vi "Keithley 2450 Digitized Sweep.vi"() -> ()   [LabVIEW 2023]
doc: "Configure the sweep with the amplitude, source settings and takes current and voltage reading.\n\nNote:\nThis VI is applicable only to 2461 model."
uses:
  Keithley 2450.lvlib
  Public/Data/Read (Multiple Points).vi
panel:
  in  "Limit Level (0.1)":dbl=0.1
  in  "Delay (0) in Sec":dbl
  in  "Sample Rate (1000Hz)":u32=2500
  in  "Sweep Points":T1={"Start "=0.0, "Stop "=5.0, "Number of Points (5)"=100}
  in  "Source Mode  (0: Voltage)":u16(ring) items=["Voltage", "Current"]
  in  "VISA resource name":refnum<visa-resource-name>
  out "Waveform Graph":dbl[][](graph)=[[-0.0001858189, 0.007417283, 0.03360542, 0.04403445, 0.04793108, 0.04931186, 0.04991157, 0.05009001, 0.050169, 0.05021289, 0.05022166, 0.0502948, 0.05017778, 0.0501924, 0.05012805, 0.05020703, 0.05027724, 0.05013097, 0.05005784, 0.05013682, 0.05028309, 0.05022166, 0.05016023, 0.05013682, 0.05026846, 0.05003736, 0.05026846, 0.05008124, 0.04967754, 0.06964044, 0.08971742, 0.09662428, 0.09915767, 0.1002605, 0.1006028, 0.1006964, 0.1009071, 0.1008047, 0.1007023, 0.1006935, 0.10079, 0.1007959, 0.1007725, 0.1007988, 0.100673, 0.1007198, 0.1008105, 0.1007052, 0.1007257, 0.1006584, 0.1006935, 0.1007754, 0.1007754, 0.1007637, 0.1007052, 0.1005882, 0.1131528, 0.1376734, 0.146435, 0.1495388, 0.1505656, 0.1511127, 0.1512063, 0.1512092, 0.1511624, 0.151139, 0.1511624, 0.1513233, 0.1511917, 0.1512999, 0.1512005, 0.151256, 0.1513321, 0.1512209, 0.1512239, 0.1510981, 0.1511624, 0.1513233, 0.1512472, 0.1512999, 0.1512999, 0.1513496, 0.151256, 0.1512999, 0.1734568, 0.1922818, 0.1985187, 0.2007771, 0.2015465, 0.2017893, 0.2019765, 0.2018595, 0.201842, 0.2017601, 0.2017893, 0.2019063, 0.2018215, 0.2016898, 0.2017103, 0.2018069], [-0.0001858189, 0.007417283, 0.03360542, 0.04403445, 0.04793108, 0.04931186, 0.04991157, 0.05009001, 0.050169, 0.05021289, 0.05022166, 0.0502948, 0.05017778, 0.0501924, 0.05012805, 0.05020703, 0.05027724, 0.05013097, 0.05005784, 0.05013682, 0.05028309, 0.05022166, 0.05016023, 0.05013682, 0.05026846, 0.05003736, 0.05026846, 0.05008124, 0.04967754, 0.06964044, 0.08971742, 0.09662428, 0.09915767, 0.1002605, 0.1006028, 0.1006964, 0.1009071, 0.1008047, 0.1007023, 0.1006935, 0.10079, 0.1007959, 0.1007725, 0.1007988, 0.100673, 0.1007198, 0.1008105, 0.1007052, 0.1007257, 0.1006584, 0.1006935, 0.1007754, 0.1007754, 0.1007637, 0.1007052, 0.1005882, 0.1131528, 0.1376734, 0.146435, 0.1495388, 0.1505656, 0.1511127, 0.1512063, 0.1512092, 0.1511624, 0.151139, 0.1511624, 0.1513233, 0.1511917, 0.1512999, 0.1512005, 0.151256, 0.1513321, 0.1512209, 0.1512239, 0.1510981, 0.1511624, 0.1513233, 0.1512472, 0.1512999, 0.1512999, 0.1513496, 0.151256, 0.1512999, 0.1734568, 0.1922818, 0.1985187, 0.2007771, 0.2015465, 0.2017893, 0.2019765, 0.2018595, 0.201842, 0.2017601, 0.2017893, 0.2019063, 0.2018215, 0.2016898, 0.2017103, 0.2018069]]
  # "(c) 2021 National Instruments.  ALL RIGHTS RESERVED."
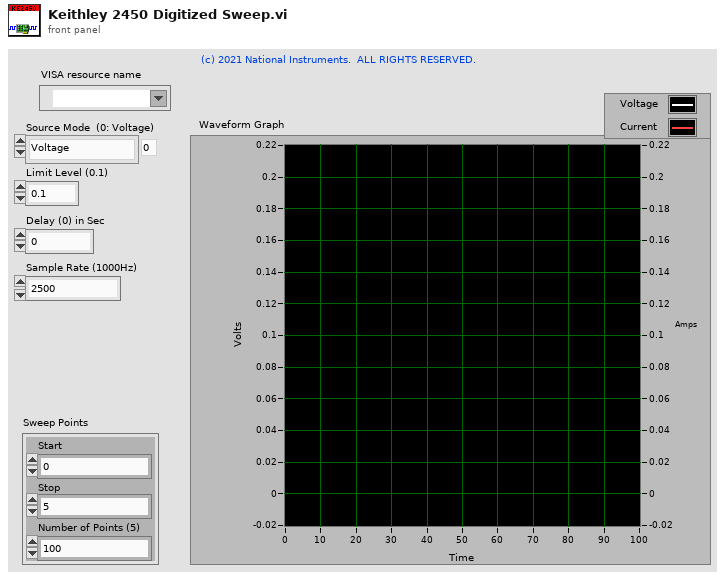
[diagram p1: front panel]
types:
  T1 = cluster{"Start ":dbl, "Stop ":dbl, "Number of Points (5)":u32}
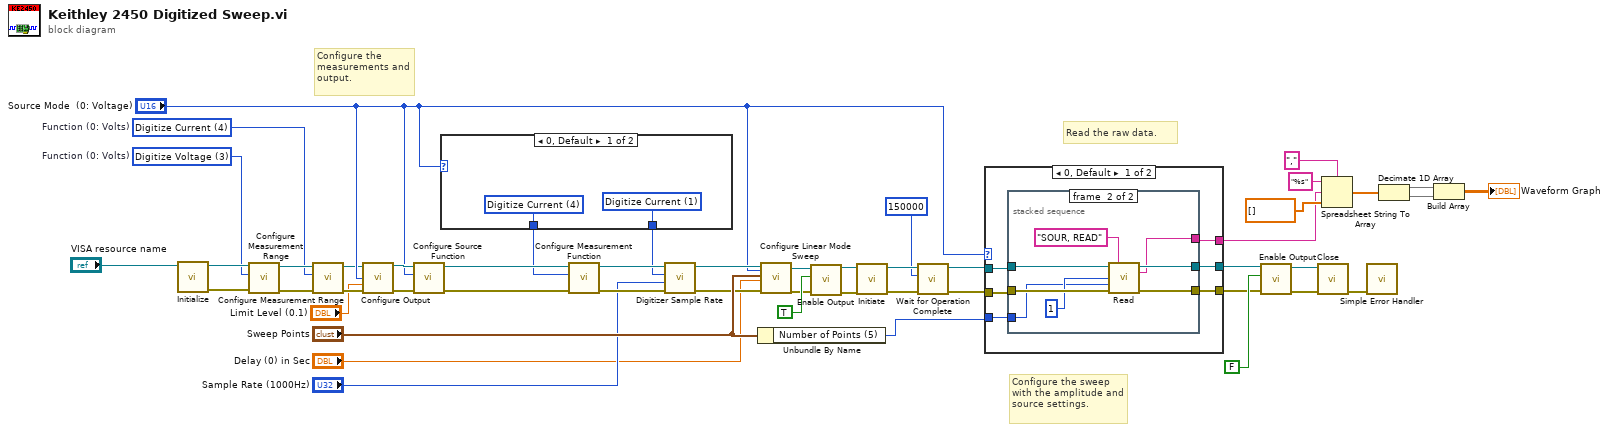
[diagram p0: block diagram]
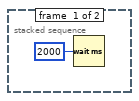
[diagram p2: hidden frame]
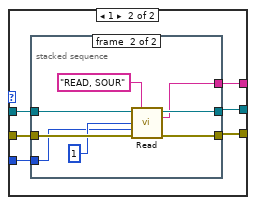
[diagram p3: hidden frame]
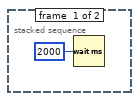
[diagram p4: hidden frame]
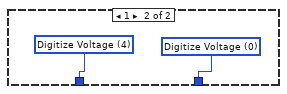
[diagram p5: hidden frame]
diagram:
  w6 = u16 4 items=["Volts", "Current", "Resistance", "Digitize Voltage", "Digitize Current"]  # Function (0: Volts)
  w7 = u16 3 items=["Volts", "Current", "Resistance", "Digitize Voltage", "Digitize Current"]  # Function (0: Volts)
  # "Read the raw data."
  # "Configure the sweep with the amplitude and source settings."
  # "Configure the measurements and output."
  n1 = call "Initialize.vi"("VISA resource name"="VISA resource name") -> ("error out"=w12:errorcluster, "VISA resource name out"=w13:refnum<visa-resource-name>)  [unwired: 9 in]
  n2 = call "Configure Measurement Range.vi"("error in (no error)"=w12, "Function (0: Volts)"=w7, "VISA resource name"=w13) -> ("error out"=w10:errorcluster, "VISA resource name out"=w11:refnum<visa-resource-name>)  [unwired: 7 in]
  n3 = call "Configure Measurement Range.vi"("error in (no error)"=w10, "Function (0: Volts)"=w6, "VISA resource name"=w11) -> ("error out"=w8:errorcluster, "VISA resource name out"=w9:refnum<visa-resource-name>)  [unwired: 7 in]
  n4 = call "Configure Output.vi"("VISA resource name"=w9, "Source Mode  (0: Voltage)"="Source Mode  (0: Voltage)", "Source Limit Level (0.1)"="Limit Level (0.1)", "error in (no error)"=w8) -> ("VISA resource name out"=w42:refnum<visa-resource-name>, "error out"=w43:errorcluster)  [unwired: 10 in]
  n5 = call "Configure Source Function.vi"("error in (no error)"=w43, "Function (0: Volts)"="Source Mode  (0: Voltage)", "VISA resource name"=w42) -> ("error out"=w25:errorcluster, "VISA resource name out"=w26:refnum<visa-resource-name>)  [unwired: 7 in]
  n6 = case shown="0, Default" "Source Mode  (0: Voltage)" {
    tunnel: [w51 w53] -> w5
    tunnel: [w50 w52] -> w4
    frame 0, Default {
      w50 = u16 1 items=["Digitize Voltage", "Digitize Current"] ("Function (0: Volts)")
      w51 = u16 4 items=["Voltage", "Current", "Resistance", "Digitize Voltage", "Digitize Current"] ("Function (0: Volts)")
    }
    frame 1 {
      w52 = u16 0 items=["Digitize Voltage", "Digitize Current"] ("Function (0: Volts)")
      w53 = u16 4 items=["Voltage", "Current", "Auto Resistance", "Manual Resistance", "Digitize Voltage", "Digitize Current"] ("Function (0: Volts)")
    }
  }
  n7 = call "Configure Measurement Function.vi"("error in (no error)"=w25, "Function (0: Volts)"=w5, "VISA resource name"=w26) -> ("error out"=w17:errorcluster, "VISA resource name out"=w18:refnum<visa-resource-name>)  [unwired: 7 in]
  n8 = call "Digitizer Sample Rate.vi"("error in (no error)"=w17, "Sample Rate (100000)"="Sample Rate (1000Hz)", "Digitize Function (Voltage)"=w4, "VISA resource name"=w18) -> ("error out"=w15:errorcluster, "VISA resource name out"=w16:refnum<visa-resource-name>)  [unwired: 6 in]
  n9 = Unbundle By Name("Sweep Points") -> ("Number of Points (5)"=w20:u32)
  n10 = call "Configure Linear Mode Sweep.vi"("VISA resource name"=w16, "Source Mode  (0: Voltage)"="Source Mode  (0: Voltage)", "Sweep Points"="Sweep Points", "Delay (0)"="Delay (0) in Sec", "error in (no error)"=w15) -> ("VISA resource name out"=w41:refnum<visa-resource-name>, "error out"=w40:errorcluster)  [unwired: 13 in]
  n11 = call "Enable Output.vi"("error in (no error)"=w40, "Enable Output (T: Enable)"=TRUE, "VISA resource name"=w41) -> ("error out"=w38:errorcluster, "VISA resource name out"=w39:refnum<visa-resource-name>)  [unwired: 7 in]
  n12 = call "Initiate.vi"("error in (no error)"=w38, "VISA resource name"=w39) -> ("error out"=w28:errorcluster, "VISA resource name out"=w29:refnum<visa-resource-name>)  [unwired: 8 in]
  n13 = call "Wait for Operation Complete.vi"("error in (no error)"=w28, "Timeout (10000 ms)"=150000, "VISA resource name"=w29) -> ("error out"=w23:errorcluster, "VISA resource name out"=w24:refnum<visa-resource-name>)  [unwired: 7 in]
  n14 = case shown="0, Default" "Source Mode  (0: Voltage)" {
    tunnel: w24 -> [w59 w74]
    tunnel: w23 -> [w58 w73]
    tunnel: [w57 w71] -> w22
    tunnel: [w56 w70] -> w21
    tunnel: w20 -> [w55 w72]
    tunnel: [w54 w69] -> w19
    frame 0, Default {
      n15 = stacked-sequence {
        tunnel: [_ w68] -> w57
        tunnel: [_ w67] -> w56
        tunnel: w59 -> [_ w65]
        tunnel: w58 -> [_ w64]
        tunnel: [_ w63] -> w54
        tunnel: w55 -> [_ w61]
        frame #0 {
          n16 = Wait (ms)(milliseconds to wait=u32 2000) -> ()  [unwired: 1 out]
        }
        frame #1 {
          n17 = call-poly "Read.vi"("VISA resource name"=w65, "Buffer Elements"="SOUR, READ", "Start Index (1)"=1, "End Index (1)"=w61, "error in (no error)"=w64) -> ("VISA resource name out"=w68:refnum<visa-resource-name>, "Data out"=w63:string, "error out"=w67:errorcluster)  [unwired: 8 in]
        }
      }
    }
    frame 1 {
      n18 = stacked-sequence {
        tunnel: [_ w83] -> w71
        tunnel: [_ w82] -> w70
        tunnel: w74 -> [_ w80]
        tunnel: w73 -> [_ w79]
        tunnel: [_ w78] -> w69
        tunnel: w72 -> [_ w76]
        frame #0 {
          n19 = Wait (ms)(milliseconds to wait=u32 2000) -> ()  [unwired: 1 out]
        }
        frame #1 {
          n20 = call-poly "Read.vi"("VISA resource name"=w80, "Buffer Elements"="READ, SOUR", "Start Index (1)"=1, "End Index (1)"=w76, "error in (no error)"=w79) -> ("VISA resource name out"=w83:refnum<visa-resource-name>, "Data out"=w78:string, "error out"=w82:errorcluster)  [unwired: 8 in]
        }
      }
    }
  }
  n21 = call "Enable Output.vi"("error in (no error)"=w21, "Enable Output (T: Enable)"=FALSE, "VISA resource name"=w22) -> ("error out"=w46:errorcluster, "VISA resource name out"=w47:refnum<visa-resource-name>)  [unwired: 7 in]
  n22 = call "Close.vi"("error in (no error)"=w46, "VISA resource name"=w47) -> ("error out"=w48:errorcluster)  [unwired: 9 in]
  n23 = Spreadsheet String To Array(delimiter (Tab)=",", format string="%s", spreadsheet string=w19, array type (2D Dbl)=dbl[] []) -> (array=w33:dbl[])
  n24 = call <vilib>:"Simple Error Handler.vi"("error in (no error)"=w48) -> ()  [unwired: 4 in, 5 out]
  n25 = Decimate 1D Array(w33) -> (w32:dbl[], w31:dbl[])
  n26 = Build Array(w32, w31) -> (→"Waveform Graph":dbl[][])
